vi "Read Attributes.vi"(11 "Random_B Msg":refnum<class "Random_B Msg.lvclass">) -> (2 "Payload":cluster{"Random":u64})   [LabVIEW 2025, in "B_Actor.lvlib" / "Random_B Msg.lvclass"]
uses:
  Random_B Msg.lvclass
  Random_B Msg.lvclass/Random_B Msg.ctl
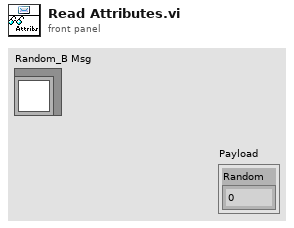
[diagram p1: front panel]
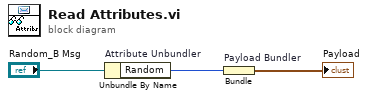
[diagram p0: block diagram]
diagram:
  n1 = Unbundle By Name "Attribute Unbundler"("Random_B Msg") -> ("Random"=w1:u64)
  n2 = Bundle "Payload Bundler"("Random"=w1) -> (→"Payload":cluster{"Random":u64})  [unwired: 1 in]
